vi "GetErrorMessageFromErrorCluster.vi"(1 "error in (no error)":errorcluster) -> (0 "trimmed string":string)   [LabVIEW 2019, in "ResultTreeListener.lvclass"]
uses:
  ResultTreeListener.lvclass
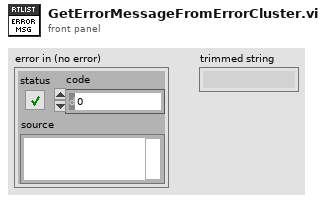
[diagram p1: front panel]
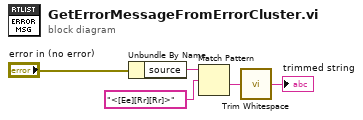
[diagram p0: block diagram]
diagram:
  n1 = Unbundle By Name("error in (no error)") -> ("source"=w5:string)
  n2 = Match Pattern(string=w5, regular expression="<[Ee][Rr][Rr]>") -> (after substring=w2:string)  [unwired: 1 in, 3 out]
  n3 = call <vilib>:"Trim Whitespace.vi"("string"=w2) -> ("trimmed string"=→"trimmed string":string)  [unwired: 1 in]
